vi "LineFollower.vi"(11 "LastNumArray":u32[](array[numeric])) -> ()   [LabVIEW 2018]
panel:
  out "array":dbl[](array[numeric])
  out "FarRight 2":bool
  out "NearRight 2":bool
  out "NearLeft 2":bool
  out "FarLeft 2":bool
  out "Center 2":bool
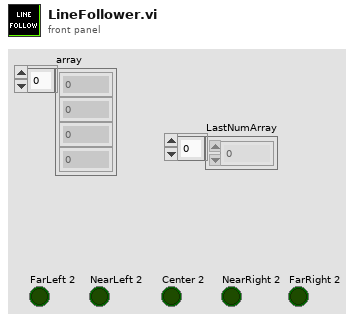
[diagram p1: front panel]
types:
  T1 = typedef "WPI_DigitalInputDevRef.ctl" = cluster{"DevStatus":errorcluster, "DIO Channel":T2}
  T2 = typedef "FPGA_DIOChannel.ctl" = enum8{"DIO 0", "DIO 1", "DIO 2", "DIO 3", "DIO 4", "DIO 5", "DIO 6", "DIO 7", "DIO 8", "DIO 9", "DIO MXP 0", "DIO MXP 1", "DIO MXP 2", "DIO MXP 3", "DIO MXP 4", "DIO MXP 5", "DIO MXP 6", "DIO MXP 7", "DIO MXP 8", "DIO MXP 9", "DIO MXP 10", "DIO MXP 11", "DIO MXP 12", "DIO MXP 13", "DIO MXP 14", "DIO MXP 15", "SPI Port CS1", "SPI Port CS2", "SPI Port CS3", "SPI Port MISO", "SPI Port MOSI", "Invalid"}
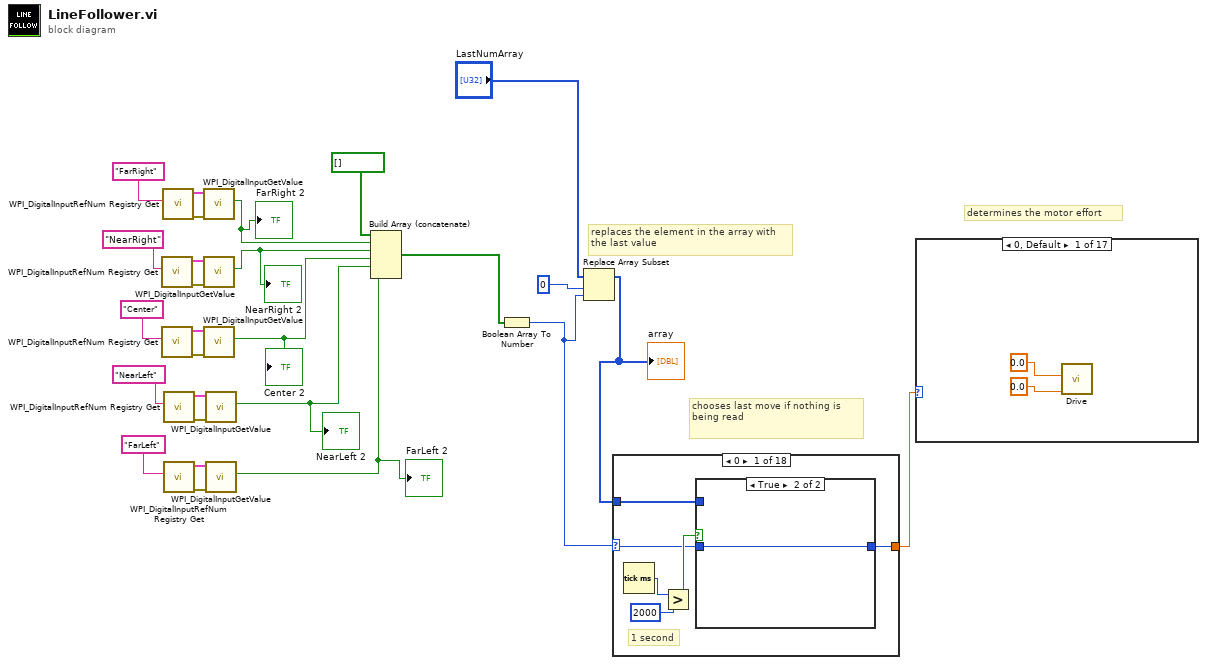
[diagram p0: block diagram]
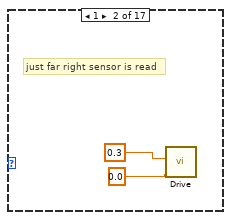
[diagram p2: hidden frame]
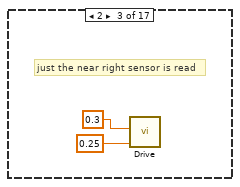
[diagram p3: hidden frame]
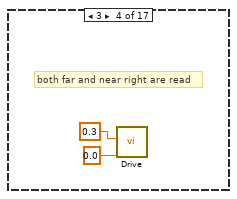
[diagram p4: hidden frame]
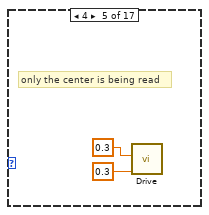
[diagram p5: hidden frame]
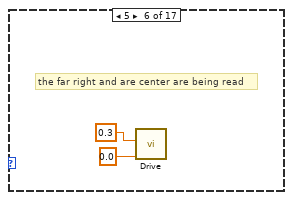
[diagram p6: hidden frame]
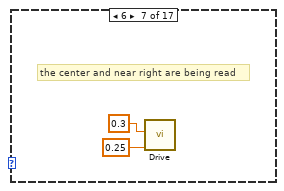
[diagram p7: hidden frame]
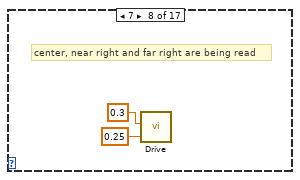
[diagram p8: hidden frame]
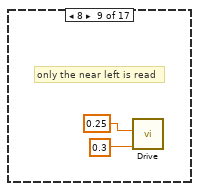
[diagram p9: hidden frame]
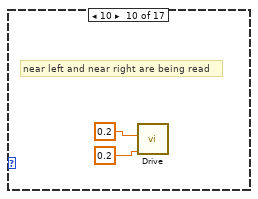
[diagram p10: hidden frame]
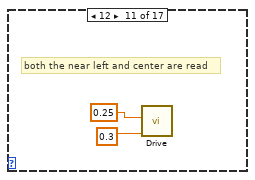
[diagram p11: hidden frame]
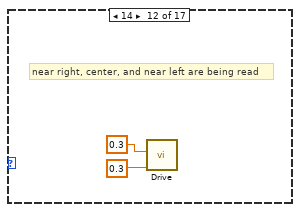
[diagram p12: hidden frame]
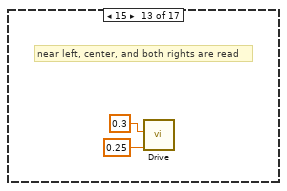
[diagram p13: hidden frame]
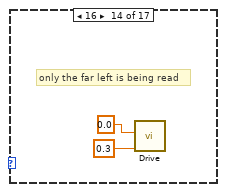
[diagram p14: hidden frame]
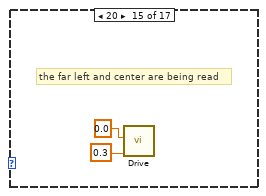
[diagram p15: hidden frame]
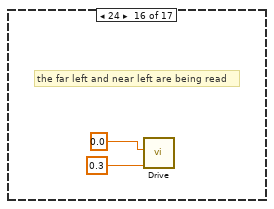
[diagram p16: hidden frame]
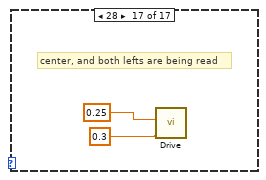
[diagram p17: hidden frame]
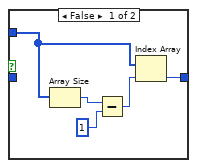
[diagram p18: hidden frame]
diagram:
  # "determines the motor effort"
  # "chooses last move if nothing is being read"
  # "replaces the element in the array with \nthe last value"
  n1 = call <vilib>:"WPI_DigitalInputRefNum Registry Get.vi"("refnum name"="NearRight") -> ("error out"=w24:errorcluster, "DigitalInputDevRef"=w23:T1)  [unwired: 9 in]
  n2 = call <vilib>:"WPI_DigitalInputRefNum Registry Get.vi"("refnum name"="Center") -> ("error out"=w21:errorcluster, "DigitalInputDevRef"=w20:T1)  [unwired: 9 in]
  n3 = call <vilib>:"WPI_DigitalInputRefNum Registry Get.vi"("refnum name"="FarRight") -> ("error out"=w27:errorcluster, "DigitalInputDevRef"=w26:T1)  [unwired: 9 in]
  n4 = call <vilib>:"WPI_DigitalInputRefNum Registry Get.vi"("refnum name"="NearLeft") -> ("error out"=w18:errorcluster, "DigitalInputDevRef"=w17:T1)  [unwired: 9 in]
  n5 = call <vilib>:"WPI_DigitalInputRefNum Registry Get.vi"("refnum name"="FarLeft") -> ("error out"=w15:errorcluster, "DigitalInputDevRef"=w14:T1)  [unwired: 9 in]
  n6 = call <vilib>:"WPI_DigitalInputGetValue.vi"("error in (no error)"=w27, "DigitalInputDevRef"=w26) -> ("Value"=w10:bool)  [unwired: 7 in, 2 out]
  "FarRight 2" <- w10
  n7 = call <vilib>:"WPI_DigitalInputGetValue.vi"("error in (no error)"=w24, "DigitalInputDevRef"=w23) -> ("Value"=w9:bool)  [unwired: 7 in, 2 out]
  "NearRight 2" <- w9
  n8 = call <vilib>:"WPI_DigitalInputGetValue.vi"("error in (no error)"=w21, "DigitalInputDevRef"=w20) -> ("Value"=w11:bool)  [unwired: 7 in, 2 out]
  "Center 2" <- w11
  n9 = call <vilib>:"WPI_DigitalInputGetValue.vi"("error in (no error)"=w18, "DigitalInputDevRef"=w17) -> ("Value"=w8:bool)  [unwired: 7 in, 2 out]
  "NearLeft 2" <- w8
  n10 = call <vilib>:"WPI_DigitalInputGetValue.vi"("error in (no error)"=w15, "DigitalInputDevRef"=w14) -> ("Value"=w7:bool)  [unwired: 7 in, 2 out]
  "FarLeft 2" <- w7
  n11 = Build Array (concatenate)(bool[] [] ("Boolean array"), w10, w9, w11, w8, w7) -> (w5:bool[])
  n12 = Boolean Array To Number(Boolean array=w5) -> (number=w4:u32)
  n13 = Replace Array Subset(array="LastNumArray", new element=w4, index=0) -> (w2:u32[])
  "array" <- w2
  n14 = case shown="0" w4 {
    selector: w4 -> [w28 w40 w41 w42 w43 w44 w45 w46 w47 w48 w49 w50 w51 w52 w53 w54 w55 _]
    tunnel: [w33 w40 w41 w42 w43 w44 w45 w46 w47 w48 w49 w50 w51 w52 w53 w54 w55 0.0 ("element")] -> w6
    tunnel: w2 -> [w32 _ _ _ _ _ _ _ _ _ _ _ _ _ _ _ _ _]
    frame 0 {
      # "1 second"
      n15 = Tick Count (ms)() -> (millisecond timer value=w31:u32)
      n16 = Greater?(x=w31, y=u32 2000) -> (0:w29:bool)
      n17 = case shown="True" w29 {
        tunnel: [w35 w39] -> w33
        tunnel: w32 -> [w34 _]
        tunnel: w28 -> [_ w39]
        frame False {
          n18 = Array Size(array=w34) -> (size(s)=w38:i32)
          n19 = Subtract(x=w38, y=1) -> (x-y=w37:i32)
          n20 = Index Array(array=w34, index=w37) -> (element=w35:u32)
        }
        frame True {
        }
      }
    }
    frame 1 {
    }
    frame 2 {
    }
    frame 3 {
    }
    frame 4 {
    }
    frame 5 {
    }
    frame 6 {
    }
    frame 7 {
    }
    frame 8 {
    }
    frame 10 {
    }
    frame 12 {
    }
    frame 14 {
    }
    frame 15 {
    }
    frame 16 {
    }
    frame 20 {
    }
    frame 24 {
    }
    frame 28 {
    }
    frame 60, Default {
      # "if it recieves a sensor value that isn't in the case structure it will return 0 or do nothing"
    }
  }
  n21 = case shown="0, Default" w6 {
    frame 0, Default {
      n22 = call "Drive.vi"("Drive R"=0.0 ("RightValue"), "Drive L"=0.0 ("LeftValue")) -> ()  [unwired: 10 in]
    }
    frame 1 {
      # "just far right sensor is read"
      n23 = call "Drive.vi"("Drive R"=0.0 ("RightValue"), "Drive L"=0.3 ("LeftValue")) -> ()  [unwired: 10 in]
    }
    frame 2 {
      # "just the near right sensor is read"
      n24 = call "Drive.vi"("Drive R"=0.25 ("RightValue"), "Drive L"=0.3 ("LeftValue")) -> ()  [unwired: 10 in]
    }
    frame 3 {
      # "both far and near right are read"
      n25 = call "Drive.vi"("Drive R"=0.0 ("RightValue"), "Drive L"=0.3 ("LeftValue")) -> ()  [unwired: 10 in]
    }
    frame 4 {
      # "only the center is being read"
      n26 = call "Drive.vi"("Drive R"=0.3 ("RightValue"), "Drive L"=0.3 ("LeftValue")) -> ()  [unwired: 10 in]
    }
    frame 5 {
      # "the far right and are center are being read"
      n27 = call "Drive.vi"("Drive R"=0.0 ("RightValue"), "Drive L"=0.3 ("LeftValue")) -> ()  [unwired: 10 in]
    }
    frame 6 {
      # "the center and near right are being read"
      n28 = call "Drive.vi"("Drive R"=0.25 ("RightValue"), "Drive L"=0.3 ("LeftValue")) -> ()  [unwired: 10 in]
    }
    frame 7 {
      # "center, near right and far right are being read"
      n29 = call "Drive.vi"("Drive R"=0.25 ("RightValue"), "Drive L"=0.3 ("LeftValue")) -> ()  [unwired: 10 in]
    }
    frame 8 {
      # "only the near left is read"
      n30 = call "Drive.vi"("Drive R"=0.3 ("RightValue"), "Drive L"=0.25 ("LeftValue")) -> ()  [unwired: 10 in]
    }
    frame 10 {
      # "near left and near right are being read"
      n31 = call "Drive.vi"("Drive R"=0.2 ("RightValue"), "Drive L"=0.2 ("LeftValue")) -> ()  [unwired: 10 in]
    }
    frame 12 {
      # "both the near left and center are read"
      n32 = call "Drive.vi"("Drive R"=0.3 ("RightValue"), "Drive L"=0.25 ("LeftValue")) -> ()  [unwired: 10 in]
    }
    frame 14 {
      # "near right, center, and near left are being read"
      n33 = call "Drive.vi"("Drive R"=0.3 ("RightValue"), "Drive L"=0.3 ("LeftValue")) -> ()  [unwired: 10 in]
    }
    frame 15 {
      # "near left, center, and both rights are read"
      n34 = call "Drive.vi"("Drive R"=0.25 ("RightValue"), "Drive L"=0.3 ("LeftValue")) -> ()  [unwired: 10 in]
    }
    frame 16 {
      # "only the far left is being read"
      n35 = call "Drive.vi"("Drive R"=0.3 ("RightValue"), "Drive L"=0.0 ("LeftValue")) -> ()  [unwired: 10 in]
    }
    frame 20 {
      # "the far left and center are being read"
      n36 = call "Drive.vi"("Drive R"=0.3 ("RightValue"), "Drive L"=0.0 ("LeftValue")) -> ()  [unwired: 10 in]
    }
    frame 24 {
      # "the far left and near left are being read"
      n37 = call "Drive.vi"("Drive R"=0.3 ("RightValue"), "Drive L"=0.0 ("LeftValue")) -> ()  [unwired: 10 in]
    }
    frame 28 {
      # "center, and both lefts are being read"
      n38 = call "Drive.vi"("Drive R"=0.3 ("RightValue"), "Drive L"=0.25 ("LeftValue")) -> ()  [unwired: 10 in]
    }
  }
